vi "Get Users With Attribute Name and Value.vi"(0 "User Configuration Manager in":refnum<class "User Configuration Manager.lvclass">, 5 "Query":T1, 11 "error in (no error)":errorcluster) -> (4 "User Configuration Manager out":refnum<class "User Configuration Manager.lvclass">, 6 "Users":string[](array[string]), 8 "Number of Users Found":u32, 15 "error out":errorcluster)   [LabVIEW 2020, in "User Configuration Manager.lvlib" / "User Configuration Manager.lvclass"]
uses:
  <vilib>/gpm_packages/@cs/user-manager/Source/User Configuration Manager/User Configuration Manager.lvclass
  <vilib>/gpm_packages/@cs/user-manager/Source/User Configuration Manager/User Configuration Manager.lvclass/User Configuration Manager.ctl
  343faba0-4591-410b-9f00-e048dfef8cf8.vi
  <vilib>/gpm_packages/@cs/user-manager/Source/User Configuration Manager/Accessors/Read Linked List Ref .vi
  <vilib>/gpm_packages/@cs/linked-list/Source/Linked List/ILinkedList/ILinked List.lvclass
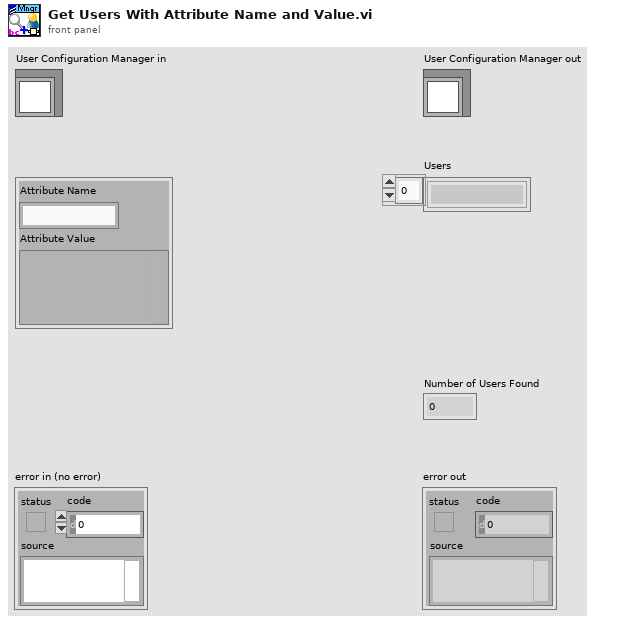
[diagram p1: front panel]
types:
  T1 = cluster{"Attribute Name":string, "Attribute Value":variant}
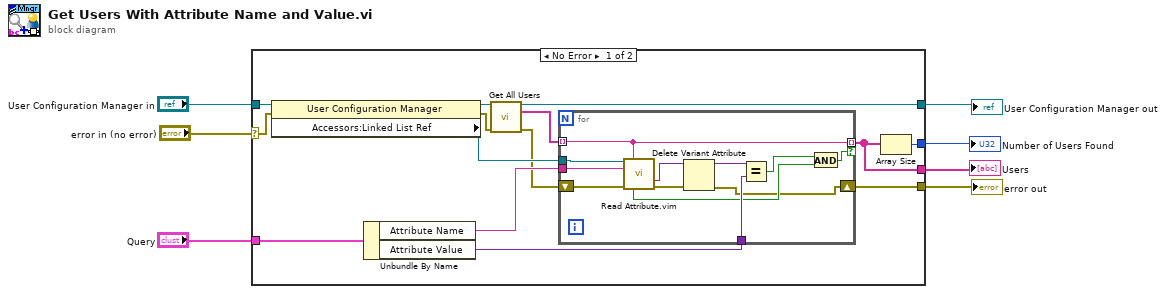
[diagram p0: block diagram]
diagram:
  n1 = case shown="No Error" "error in (no error)" {
    selector: "error in (no error)" -> [w13 w34]
    tunnel: "User Configuration Manager in" -> [w19 w35]
    tunnel: [w11 w35] -> w5
    tunnel: "Query" -> [w18 _]
    tunnel: [w14 w34] -> w3
    tunnel: [w21 _] -> w2
    tunnel: [w15 _] -> w1
    frame No Error {
      n2 = property class="User Configuration Manager"(reference=w19, error in=w13) -> (reference out=w12:refnum<class "User Configuration Manager.lvclass">, error out=w9:errorcluster, "Accessors:Linked List Ref "=w20:refnum<data-value>)
      n3 = Unbundle By Name(w18) -> ("Attribute Name"=w17:string, "Attribute Value"=w16:variant)
      n4 = call-dynamic "Get All Users.vi"("User Configuration Manager in"=w12, "error in (no error)"=w9) -> ("User Configuration Manager out"=w11:refnum<class "User Configuration Manager.lvclass">, "Users"=w10:string[], "error out"=w8:errorcluster)  [unwired: 10 in, 1 out]
      n5 = for {
        tunnel: w20 -> [w33]
        tunnel: w10 -> [w31] mode=indexing
        tunnel: w17 -> [w32]
        tunnel: [w31] -> w15 mode=indexing if=w28
        shift-right: [w22] -> w14
        shift-left: w8 -> [w30]
        tunnel: w16 -> [w29]
        n6 = call "Read Attribute.vim"("Linked List Ref"=w33, "Linked List ID"=w31, "Attribute Name"=w32, "error in (no error)"=w30) -> ("Attribute"=w25:variant, "Found?"=w27:bool, "error out"=w23:errorcluster)  [unwired: 6 in, 3 out]
        n7 = Delete Variant Attribute(4:w23, 7:w25) -> (0:w22:errorcluster, 3:w24:variant)  [unwired: 1 in, 1 out]
        n8 = Equal?(x=w24, y=w29) -> (x = y?=w26:bool)
        n9 = And(x=w26, y=w27) -> (x .and. y?=w28:bool)
      }
      n10 = Array Size(array=w15) -> (size(s)=w21:i32)
    }
    frame Error {
    }
  }
  "error out" <- w3
  "User Configuration Manager out" <- w5
  "Users" <- w1
  "Number of Users Found" <- w2
